vi "表格数据转化为数组.vi"(11 "标定点数":string[][](table)) -> (1 "limit":cluster{dbl[], dbl[], dbl[]}, 2 "未补偿0数组":dbl[][](array[numeric]), 3 "补偿0数组":dbl[](array[numeric]))   [LabVIEW 2019]
panel:
  out "初始化的数组":dbl[](array[numeric])
  out "数组 4":dbl[](array[numeric])
  out "子数组 3":string[](array[string])
  out "数组 3":dbl[](array[numeric])
  out "子数组 2":string[](array[string])
  out "子数组":string[](array[string])
  out "数组 2":dbl[](array[numeric])
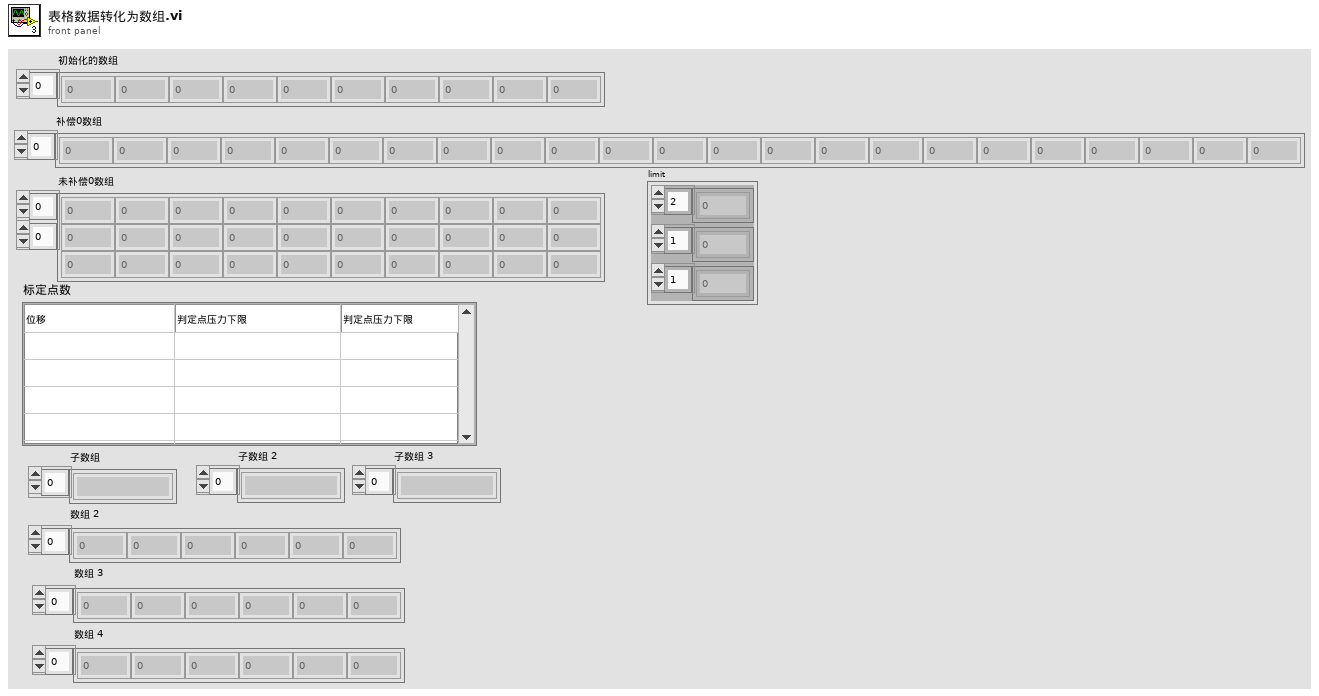
[diagram p1: front panel]
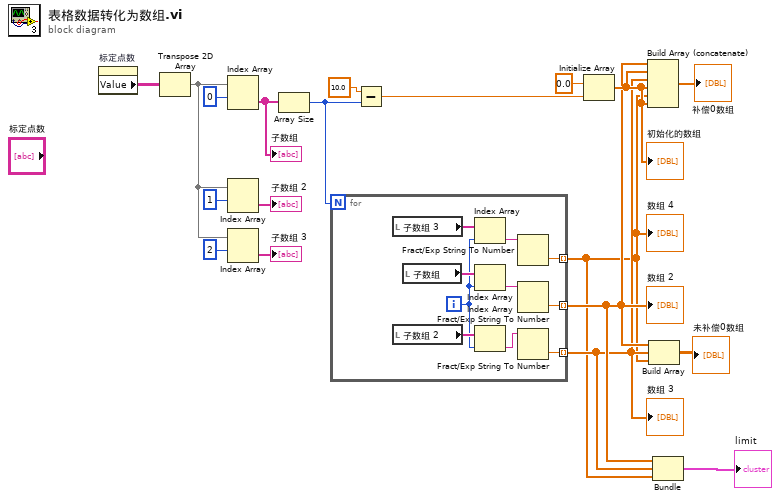
[diagram p0: block diagram]
diagram:
  n1 = property on="标定点数" class="Tbl (严格)"() -> ("Value"=w17:string[][])  [unwired: 2 in, 2 out]
  n2 = Transpose 2D Array(2D array=w17) -> (transposed array=w14:string[][])
  n3 = Index Array(array=w14, index (row)=0 ("索引 (行)")) -> (element=w18:string[])  [unwired: 1 in]
  "子数组" <- w18
  n4 = Index Array(array=w14, index (row)=1 ("索引 (行)")) -> (element=→"子数组 2":string[])  [unwired: 1 in]
  n5 = Index Array(array=w14, index (row)=2 ("索引 (行)")) -> (element=→"子数组 3":string[])  [unwired: 1 in]
  n6 = Array Size(array=w18) -> (size(s)=w8:i32)
  n7 = for {
    N: w8 -> [_]
    tunnel: [w27] -> w3 mode=indexing
    tunnel: [w24] -> w2 mode=indexing
    tunnel: [w20] -> w1 mode=indexing
    i -> [w22]
    n8 = local read "子数组 3"() -> (w23:string[])
    n9 = local read "子数组 2"() -> (w26:string[])
    n10 = local read "子数组"() -> (w29:string[])
    n11 = Index Array(array=w23, index=w22) -> (element=w21:string)
    n12 = Index Array(array=w29, index=w22) -> (element=w28:string)
    n13 = Index Array(array=w26, index=w22) -> (element=w25:string)
    n14 = Fract/Exp String To Number(string=w21) -> (number=w20:dbl)  [unwired: 3 in, 1 out]
    n15 = Fract/Exp String To Number(string=w28) -> (number=w27:dbl)  [unwired: 3 in, 1 out]
    n16 = Fract/Exp String To Number(string=w25) -> (number=w24:dbl)  [unwired: 3 in, 1 out]
  }
  "数组 2" <- w3
  "数组 3" <- w2
  "数组 4" <- w1
  n17 = Subtract(x=10.0, y=w8) -> (x-y=w7:dbl)
  n18 = Initialize Array(0.0 ("元素"), w7) -> (w6:dbl[])
  "初始化的数组" <- w6
  n19 = Build Array (concatenate)(w3, w6, w2, w6, w1, w6) -> (→"补偿0数组":dbl[])
  n20 = Build Array(w3, w2, w1) -> (→"未补偿0数组":dbl[][])
  n21 = Bundle(w3, w2, w1) -> (→"limit":cluster{dbl[], dbl[], dbl[]})  [unwired: 1 in]
